vi "_Read.vi"(8 "error in (no error)":errorcluster, 11 "Power Meter in":refnum<class "Power Meter.lvclass">) -> (0 "error out":errorcluster, 2 "X array":T1, 3 "Power Meter out":refnum<class "Power Meter.lvclass">)   [LabVIEW 2009, in "Power Meter.lvclass"]
doc: "(Protected, Dynamic, Pure Virtual/Abstract) Perform a measurement and return one or more channels of data. Outsiders should not call this method, but instead the public \"Read Data.vi\"."
uses:
  Power Meter.lvclass
  Utility Classes/Readable/X array.ctl
  Utility Classes/Readable/X.ctl
  Utility Classes/Readable/Readable.lvclass
  Newport 1830-C/Newport 1830-C.lvlib
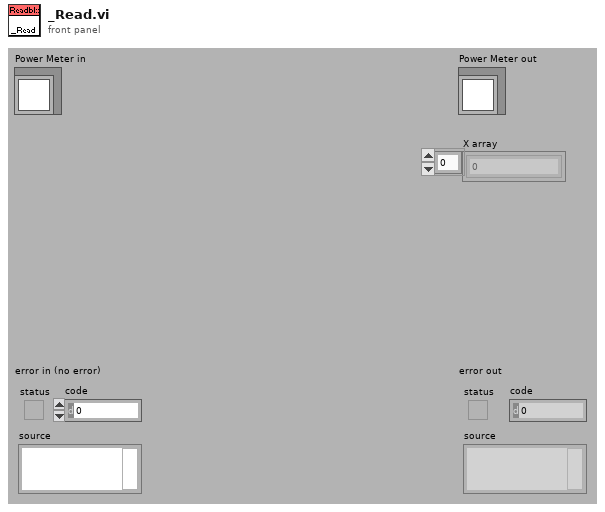
[diagram p1: front panel]
types:
  T1 = typedef "Readable.lvclass/X array.ctl" = T2[]
  T2 = typedef "Readable.lvclass/X.ctl" = dbl
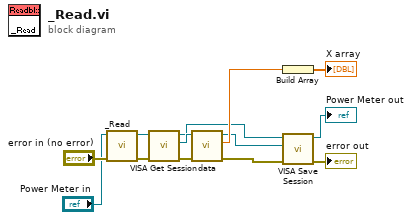
[diagram p0: block diagram]
diagram:
  n1 = call-parent "_Read.vi"("error in (no error)"="error in (no error)", "Readable in"="Power Meter in") -> ("error out"=w6:errorcluster, "Readable out"=w11:refnum<class "Power Meter.lvclass">)  [unwired: 7 in, 1 out]
  n2 = call-dynamic "VISA Get Session.vi"("error in (no error)"=w6, "Instrument.lvclass in"=w11) -> ("error out"=w7:errorcluster, "VISA Resource Name"=w10:refnum<visa-resource-name>, "Instrument.lvclass out"=w4:refnum<class "Power Meter.lvclass">)  [unwired: 7 out]
  n3 = call "data.vi"("error in (no error)"=w7, "VISA resource name"=w10) -> ("error out"=w2:errorcluster, "output"=w9:dbl, "VISA resource name out"=w5:refnum<visa-resource-name>)  [unwired: 6 in, 1 out]
  n4 = Build Array(w9) -> (→"X array":dbl[])
  n5 = call-dynamic "VISA Save Session.vi"("error in (no error)"=w2, "VISA Resource Name"=w5, "Instrument.lvclass in"=w4) -> ("error out"=→"error out":errorcluster, "Instrument.lvclass out"=→"Power Meter out":refnum<class "Power Meter.lvclass">)  [unwired: 7 out]
